vi "convert sensor voltage to real measurements.vi"(9 "Input Variables and Slopes":T2={"Total Volume"=0.0, "String Pot Slope"=0.0, "Flow Slope"=0.0, "Up Hole Pressure Slope"=0.0, "Depth to Water Table"=0.0, "Atmospheric Pressure"=0.0, "Reservoir Pressure"=0.0, "Height of Sample Box"=0.0, "DH Pressure Trans Slope"=0.0, "DH Pressure Offset"=0.0, "Up Hole  Pressure Offset"=0.0, "Aux 1 Slope"=1.6619999408721924, "Aux 2 Slope"=39.040000915527344, "Aux 3 Slope"=48.27000045776367} {"Aux 3 Slope" format="%.2f"; "Aux 2 Slope" format="%.2f"; "Aux 1 Slope" format="%.2f"; "Up Hole  Pressure Offset" format="%.2f"; "DH Pressure Offset" format="%.2f"; "DH Pressure Trans Slope" format="%.2f"; "Height of Sample Box" format="%.2f"; "Reservoir Pressure" format="%.2f"; "Atmospheric Pressure" format="%.2f"; "Depth to Water Table" format="%.2f"; "Up Hole Pressure Slope" format="%.2f"; "Flow Slope" format="%.2f"; "String Pot Slope" format="%.2f"; "Total Volume" format="%.2f"}, 10 "Sensor  Real Measurements in":T1, 11 "Sensor Cluster":T1) -> (3 "Sensor  Real Measurements out":T1)   [LabVIEW 2016]
uses:
  controls/MCC DAQ Readings.ctl
  Control 2.ctl
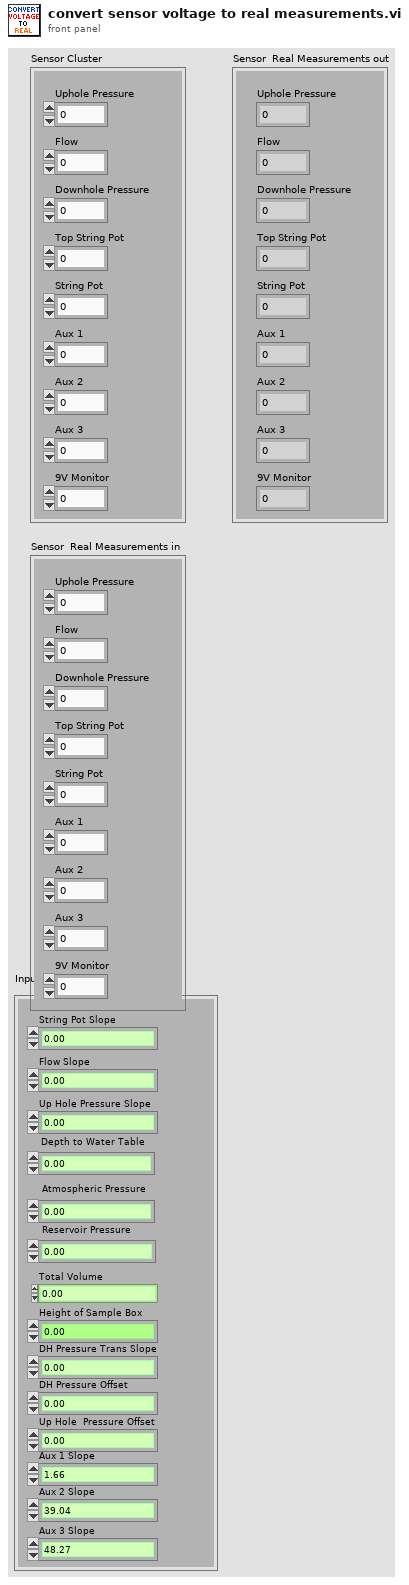
[diagram p1: front panel]
types:
  T1 = typedef "MCC DAQ Readings.ctl" = cluster{"Uphole Pressure":dbl, "Flow":dbl, "Downhole Pressure":dbl, "Top String Pot":dbl, "String Pot":dbl, "Aux 1":dbl, "Aux 2":dbl, "Aux 3":dbl, "9V Monitor":dbl}
  T2 = typedef "Control 2.ctl" = cluster{"Total Volume":dbl, "String Pot Slope":dbl, "Flow Slope":dbl, "Up Hole Pressure Slope":dbl, "Depth to Water Table":dbl, "Atmospheric Pressure":dbl, "Reservoir Pressure":dbl, "Height of Sample Box":dbl, "DH Pressure Trans Slope":dbl, "DH Pressure Offset":dbl, "Up Hole  Pressure Offset":dbl, "Aux 1 Slope":dbl, "Aux 2 Slope":dbl, "Aux 3 Slope":dbl}
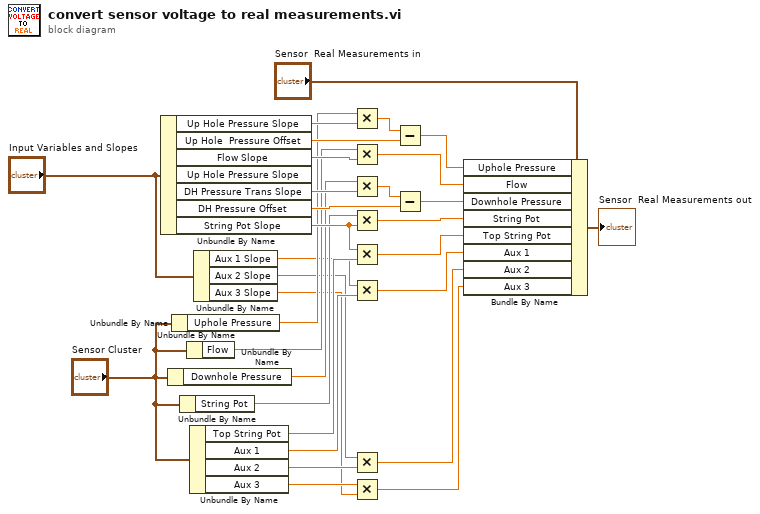
[diagram p0: block diagram]
diagram:
  n1 = Unbundle By Name("Input Variables and Slopes") -> ("Up Hole Pressure Slope"=w14:dbl, "Up Hole  Pressure Offset"=w17:dbl, "Flow Slope"=w19:dbl, "DH Pressure Trans Slope"=w22:dbl, "DH Pressure Offset"=w24:dbl, "String Pot Slope"=w28:dbl)  [unwired: 1 out]
  n2 = Unbundle By Name("Sensor Cluster") -> ("Downhole Pressure"=w21:dbl)
  n3 = Unbundle By Name("Sensor Cluster") -> ("Uphole Pressure"=w13:dbl)
  n4 = Unbundle By Name("Sensor Cluster") -> ("String Pot"=w26:dbl)
  n5 = Unbundle By Name("Sensor Cluster") -> ("Flow"=w18:dbl)
  n6 = Unbundle By Name("Sensor Cluster") -> ("Top String Pot"=w29:dbl, "Aux 1"=w10:dbl, "Aux 2"=w9:dbl, "Aux 3"=w8:dbl)
  n7 = Unbundle By Name("Input Variables and Slopes") -> ("Aux 1 Slope"=w3:dbl, "Aux 2 Slope"=w2:dbl, "Aux 3 Slope"=w1:dbl)
  n8 = Multiply(x=w13, y=w14) -> (x*y=w16:dbl)
  n9 = Multiply(x=w18, y=w19) -> (x*y=w20:dbl)
  n10 = Multiply(x=w21, y=w22) -> (x*y=w23:dbl)
  n11 = Multiply(x=w26, y=w28) -> (x*y=w27:dbl)
  n12 = Multiply(x=w28, y=w29) -> (x*y=w30:dbl)
  n13 = Multiply(x=w3, y=w10) -> (x*y=w7:dbl)
  n14 = Multiply(x=w2, y=w9) -> (x*y=w6:dbl)
  n15 = Multiply(x=w8, y=w1) -> (x*y=w5:dbl)
  n16 = Subtract(x=w16, y=w17) -> (x-y=w15:dbl)
  n17 = Subtract(x=w23, y=w24) -> (x-y=w25:dbl)
  n18 = Bundle By Name(cluster="Sensor  Real Measurements in", "Uphole Pressure"=w15, "Flow"=w20, "Downhole Pressure"=w25, "String Pot"=w27, "Top String Pot"=w30, "Aux 1"=w7, "Aux 2"=w6, "Aux 3"=w5) -> (→"Sensor  Real Measurements out":T1)
